vi "Motor_OpenSendRead.vi"(11 "Angle to move":dbl=-1.0) -> (0 "error out":errorcluster, 2 "steps":i32, 3 "reply":string)   [LabVIEW 2022 SP3]
panel:
  out "Timeouts":bool[](array[boolean])
  # "Note:  angle = -1 does a tap"
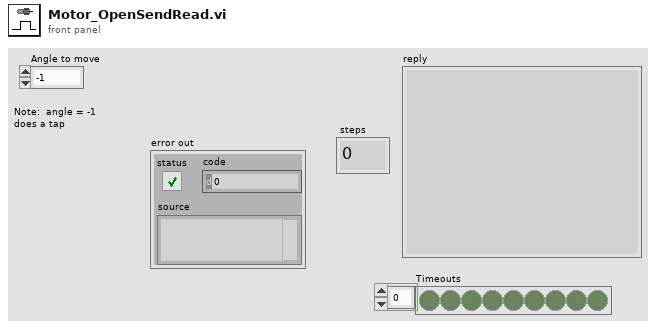
[diagram p1: front panel]
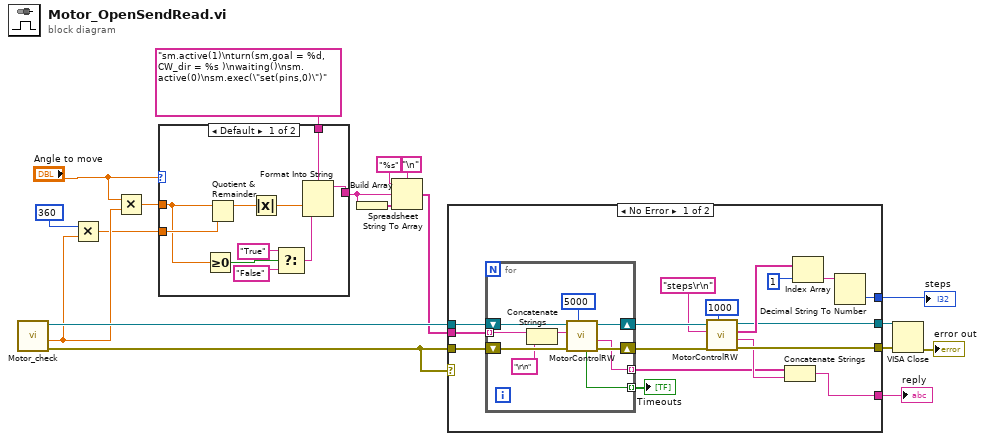
[diagram p0: block diagram]
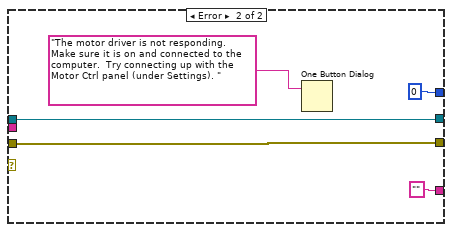
[diagram p2: hidden frame]
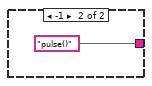
[diagram p3: hidden frame]
diagram:
  n1 = call "Motor_check.vi"() -> ("error out"=w15:errorcluster, "steps per degree out"=w2:dbl, "VISA Refnum out"=w18:refnum<visa-resource-name>)  [unwired: 8 in, 1 out]
  n2 = Multiply(x=u32 360, y=w2) -> (x*y=w1:dbl)
  n3 = Multiply(x="Angle to move", y=w2) -> (x*y=w5:dbl)
  n4 = case shown="Default" "Angle to move" {
    tunnel: [w28 "pulse()" ("element")] -> w9
    tunnel: w5 -> [w21 _]
    tunnel: "sm.active(1)\nturn(sm,goal = %d, CW_dir = %s )\nwaiting()\nsm.active(0)\nsm.exec(\"set(pins,0)\")" ("element") -> [w27 _]
    tunnel: w1 -> [w22 _]
    frame Default {
      n5 = Greater Or Equal To 0?(x=w21) -> (x >= 0?=w26:bool)
      n6 = Quotient & Remainder(x=w21, y=w22) -> (x-y*floor(x/y)=w20:dbl)  [unwired: 1 out]
      n7 = Absolute Value(x=w20) -> (abs(x)=w19:dbl)
      n8 = Select(t="True" ("format string"), s=w26, f="False" ("format string")) -> (s? t:f=w23:string)
      n9 = Format Into String(format string=w27, w19, w23) -> (resulting string=w28:string)  [unwired: 2 in, 1 out]
    }
    frame -1 {
    }
  }
  n10 = Build Array(w9) -> (w8:string[])
  n11 = Spreadsheet String To Array(delimiter (Tab)="\n", format string="%s", spreadsheet string=w9, array type (2D Dbl)=w8) -> (array=w10:string[])
  n12 = case shown="No Error" w15 {
    tunnel: w18 -> [w46 w57]
    tunnel: w15 -> [w45 w60]
    tunnel: w10 -> [w31 _]
    tunnel: [w35 w60] -> w12
    tunnel: [w37 0] -> w17
    tunnel: [w33 "" ("reply")] -> w16
    tunnel: [w36 w57] -> w14
    frame No Error {
      n13 = for {
        shift-right: [w53] -> w41
        shift-left: w46 -> [w56]
        shift-right: [w54] -> w42
        shift-left: w45 -> [w55]
        tunnel: [w51] -> w32 mode=indexing
        tunnel: w31 -> [w50] mode=indexing
        tunnel: [w47] -> w30 mode=indexing
        n14 = Concatenate Strings(w50, "\r\n" ("element")) -> (w48:string)
        n15 = call "MotorControlRW.vi"("timeout (msec)"=u32 5000, "error in (no error)"=w55, "payload"=w48, "VISA in"=w56) -> ("error out"=w54:errorcluster, "reply"=w51:string, "VISA Out"=w53:refnum<visa-resource-name>, "Timed out"=w47:bool)  [unwired: 3 in, 1 out]
      }
      "Timeouts" <- w30
      n16 = call "MotorControlRW.vi"("timeout (msec)"=u32 1000, "error in (no error)"=w42, "payload"="steps\r\n" ("element"), "VISA in"=w41) -> ("error out"=w35:errorcluster, "reply"=w34:string, "rows"=w39:string[], "VISA Out"=w36:refnum<visa-resource-name>)  [unwired: 3 in, 1 out]
      n17 = Concatenate Strings(w32, w34) -> (w33:string)
      n18 = Index Array(array=w39, index=1) -> (element=w44:string)
      n19 = Decimal String To Number(string=w44) -> (number=w37:i32)  [unwired: 2 in, 1 out]
    }
    frame Error {
      n20 = One Button Dialog(message="The motor driver is not responding.  Make sure it is on and connected to the computer.  Try connecting up with the Motor Ctrl panel (under Settings). ") -> ()  [unwired: 1 in, 1 out]
    }
  }
  "steps" <- w17
  "reply" <- w16
  n21 = VISA Close(VISA resource name=w14, error in (no error)=w12) -> (error out=→"error out":errorcluster)
